vi "Write All Stderr.vi"(8 "Error In":errorcluster, 10 "Data":u8[](array[numeric]), 11 "Channel In":refnum<class "Channel.lvclass">) -> (0 "Error Out":errorcluster, 2 "Write Count":u64, 3 "Channel Out":refnum<class "Channel.lvclass">)   [LabVIEW 2018, in "Toolkit.lvlib" / "Channel.lvclass"]
doc: "Writes binary data to the STDERR stream of the SSH channel represented by this Channel object until all of the data (bytes) are written. If the binary data is larger than 30KB, then the data is written in 30KB chunks, or blocks, until the <B>Write Count</B> equals the <B>Data</B> array size."
uses:
  Channel.lvclass
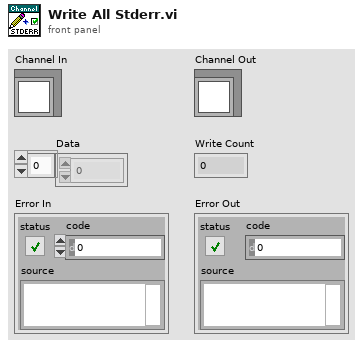
[diagram p1: front panel]
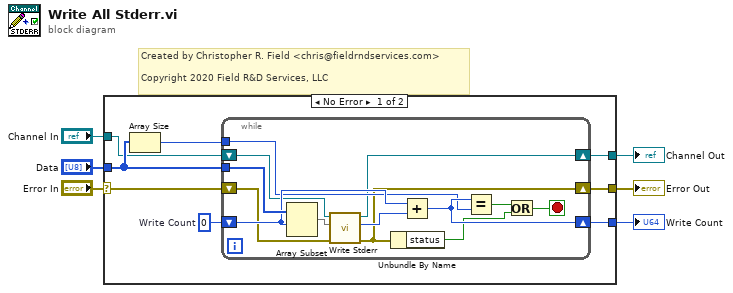
[diagram p0: block diagram]
diagram:
  # "Created by Christopher R. Field <chris@fieldrndservices.com>\n\nCopyright 2020 Field R&D Services, LLC"
  n1 = case shown="No Error" "Error In" {
    selector: "Error In" -> [w8 w28]
    tunnel: "Data" -> [w12 _]
    tunnel: "Channel In" -> [w11 w29]
    tunnel: [w10 w29] -> w4
    tunnel: [w9 w28] -> w3
    tunnel: [w7 _] -> w1
    frame No Error {
      w13 = u64 0  # Write Count
      n2 = Array Size(array=w12) -> (size(s)=w14:i32)
      n3 = while {
        tunnel: w12 -> [w27]
        shift-right: [w17] -> w9
        shift-left: w8 -> [w16]
        shift-right: [w19] -> w10
        shift-left: w11 -> [w20]
        tunnel: w14 -> [w24]
        shift-right: [w25] -> w7
        shift-left: w13 -> [w26]
        stop <- w21 stop-if-true
        n4 = Array Subset(array=w27, index=w26) -> (w15:u8[])  [unwired: 1 in]
        n5 = call "Write Stderr.vi"("Error In"=w16, "Data"=w15, "Channel In"=w20) -> ("Error Out"=w17:errorcluster, "Write Count"=w18:u64, "Channel Out"=w19:refnum<class "Channel.lvclass">)  [unwired: 6 in]
        n6 = Unbundle By Name(w17) -> ("status"=w22:bool)
        n7 = Add(x=w26, y=w18) -> (x+y=w25:u64)
        n8 = Equal?(x=w25, y=w24) -> (x = y?=w23:bool)
        n9 = Or(x=w23, y=w22) -> (x .or. y?=w21:bool)
      }
    }
    frame Error {
    }
  }
  "Channel Out" <- w4
  "Error Out" <- w3
  "Write Count" <- w1
